vi "piechart.vi"(7 "Pie Chart Size":i16=200, 8 "Colors":u32[](array[colorbox])=[11796480, 37103, 40712, 16770816, 11796658, 4210752], 9 "Values":dbl[](array[numeric])=[7.0, 5.0, 12.0, 4.0, 3.0, 4.0] format="%.2f") -> (2 "Percent %":dbl[](array[numeric]) format="%.2f", 3 "Pie Chart":picture)   [LabVIEW 2014]
panel:
  # "This VI demonstrates how to create a pie chart in LabVIEW.\nRun the VI and notice that LabVIEW draws the pie chart and populates the percent fields.\nAdd your own values to change the percentage and modify the pie chart. You also can modify\nthe pie chart size."
  # "Legend"
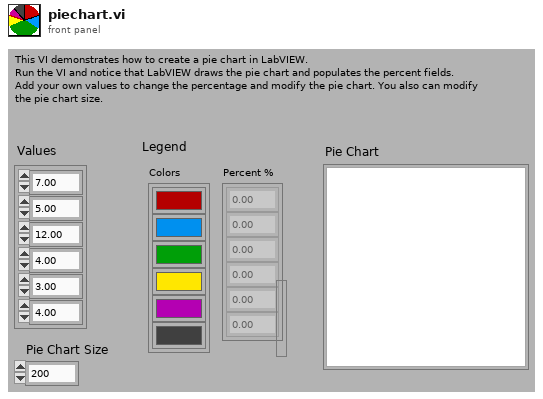
[diagram p1: front panel]
types:
  T1 = cluster{"left":i16, "top":i16, "right":i16, "bottom":i16}
  T2 = cluster{"Pie Chart Size":i16, "Pie Chart Size":i16}
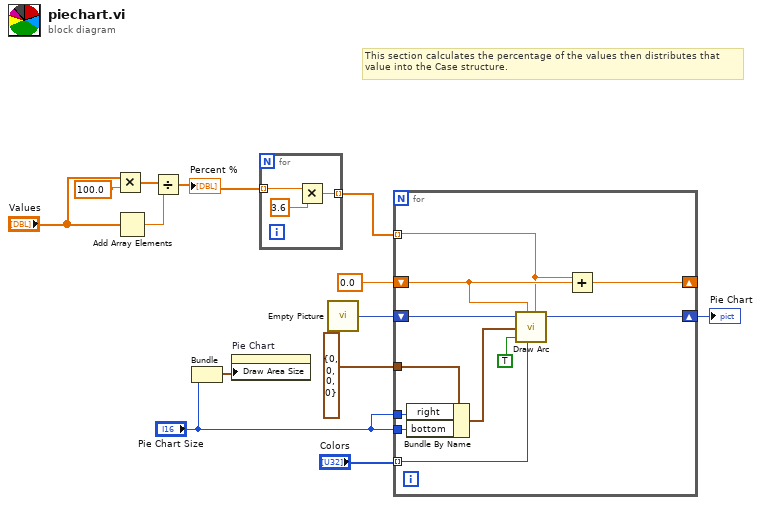
[diagram p0: block diagram]
diagram:
  # "This section calculates the percentage of the values then distributes that\nvalue into the Case structure."
  n1 = Multiply(x="Values", y=100.0) -> (x*y=w8:dbl[])
  n2 = Add Array Elements(numeric array="Values") -> (sum=w5:dbl)
  n3 = Divide(x=w8, y=w5) -> (x/y=w4:dbl[])
  "Percent %" <- w4
  n4 = Bundle("Pie Chart Size"="Pie Chart Size", "Pie Chart Size"="Pie Chart Size") -> (w3:T2)  [unwired: 1 in]
  n5 = property on="Pie Chart" class="Pict"("Draw Area Size"=w3) -> ()  [unwired: 2 in, 2 out]
  n6 = for {
    tunnel: w4 -> [w15] mode=indexing
    tunnel: [w16] -> w7 mode=indexing
    n7 = Multiply(x=w15, y=3.6) -> (x*y=w16:dbl)
  }
  n8 = call "Empty Picture"() -> ("empty picture"=w11:picture)
  n9 = for {
    shift-right: [w26] -> w13
    shift-left: w11 -> [w27]
    shift-right: [w21] -> _
    shift-left: 0.0 -> [w24]
    tunnel: "Colors" -> [w23] mode=indexing
    tunnel: w7 -> [w22] mode=indexing
    tunnel: "Pie Chart Size" -> [w20]
    tunnel: "Pie Chart Size" -> [w19]
    tunnel: T1 {"left"=0, "top"=0, "right"=0, "bottom"=0} ("rect") -> [w18]
    n10 = Bundle By Name(cluster=w18, "right"=w20, "bottom"=w19) -> (w17:T1)
    n11 = call <vilib>:"Draw Arc.vi"("picture"=w27, "start angle[degrees]"=w24, "rect"=w17, "fill?(F)"=TRUE, "color(black)"=w23, "arc size[degrees]"=w22) -> ("new picture"=w26:picture)  [unwired: 3 in]
    n12 = Add(x=w22, y=w24) -> (x+y=w21:dbl)
  }
  "Pie Chart" <- w13
